vi "ActDriveStraightCommon.vi"(10 "FirstTime":bool, 11 "Dist (ft)":dbl) -> (3 "Error":dbl)   [LabVIEW 2020]
uses:
  <vilib>/Rock Robotics/Network Tables/NT Write Boolean.vi
  <vilib>/Rock Robotics/Network Tables/NT Write Number.vi
  <vilib>/Rock Robotics/Network Tables/NT Write Numeric Array.vi
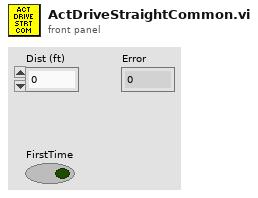
[diagram p1: front panel]
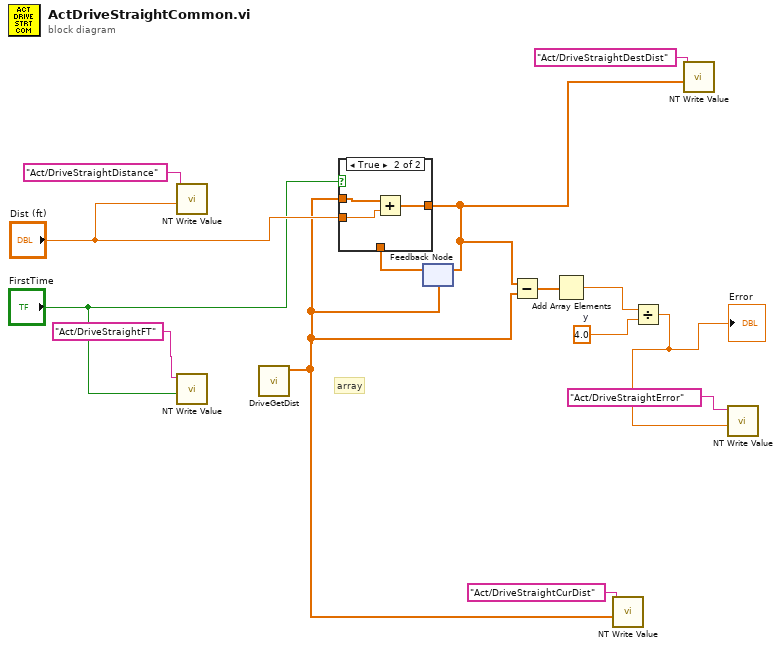
[diagram p0: block diagram]
diagram:
  w7 = 4.0  # y
  # "array"
  n1 = call-poly <vilib>:"NT Write Value.vi"("value"="Dist (ft)", "name"="Act/DriveStraightDistance") -> ()  [unwired: 9 in, 1 out]
  n2 = call-poly <vilib>:"NT Write Value.vi"("value"="FirstTime", "name"="Act/DriveStraightFT") -> ()  [unwired: 9 in, 1 out]
  n3 = call "DriveGetDist.vi"() -> ("ModuleTravelPosition"=w1:dbl[])  [unwired: 11 in]
  n4 = feedback #1(w1) -> (w13:dbl[])
  n5 = case shown="True" "FirstTime" {
    tunnel: "Dist (ft)" -> [_ w17]
    tunnel: w1 -> [_ w18]
    tunnel: [w15 w16] -> w3
    tunnel: w13 -> [w15 _]
    frame False {
    }
    frame True {
      n6 = Add(x=w18, y=w17) -> (x+y=w16:dbl[])
    }
  }
  n7 = feedback-in #1(w3) -> ()
  n8 = Subtract(x=w3, y=w1) -> (x-y=w14:dbl[])
  n9 = Add Array Elements(numeric array=w14) -> (sum=w6:dbl)
  n10 = call-poly <vilib>:"NT Write Value.vi"("value"=w1, "name"="Act/DriveStraightCurDist") -> ()  [unwired: 9 in, 1 out]
  n11 = Divide(x=w6, y=w7) -> (x/y=w5:dbl)
  "Error" <- w5
  n12 = call-poly <vilib>:"NT Write Value.vi"("value"=w3, "name"="Act/DriveStraightDestDist") -> ()  [unwired: 9 in, 1 out]
  n13 = call-poly <vilib>:"NT Write Value.vi"("value"=w5, "name"="Act/DriveStraightError") -> ()  [unwired: 9 in, 1 out]
